vi "create temp folder.vi"(8 "error in":errorcluster, 9 "Temp?":bool, 11 "Path in":path) -> (0 "error out":errorcluster, 3 "Path out":path)   [LabVIEW 2023, in "User Interface.lvlib"]
uses:
  User Interface.lvlib
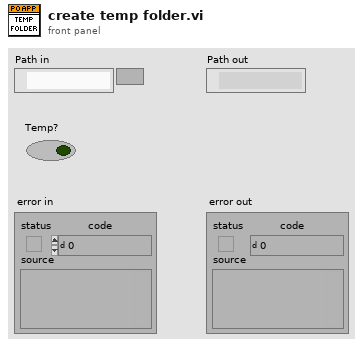
[diagram p1: front panel]
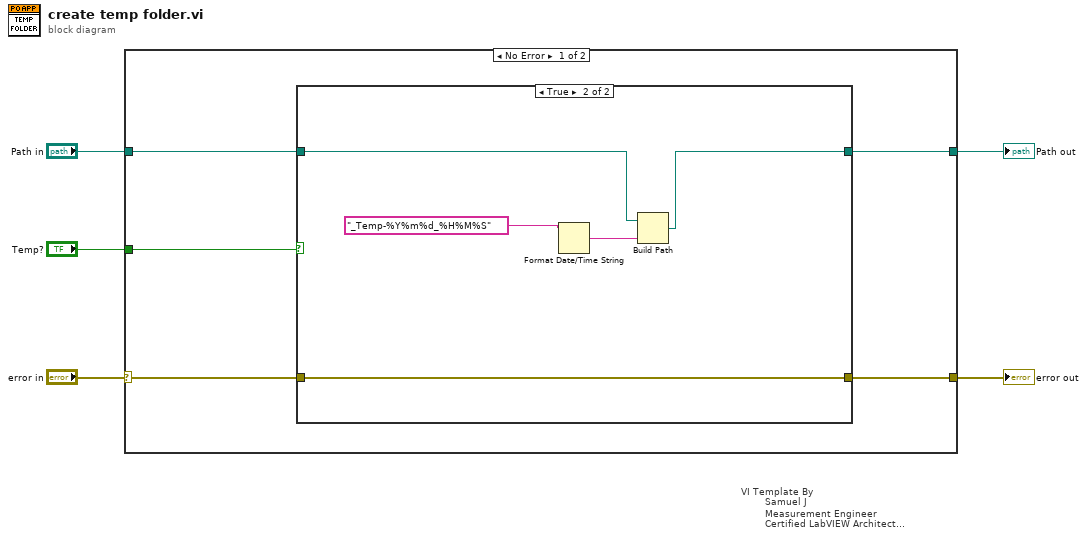
[diagram p0: block diagram]
diagram:
  n1 = case "VI Template By\n        Samuel J\n        Measurement Engineer\n        Certified LabVIEW Architect\n        Vestas Technology R&D Chennai" shown="No Error" "error in" {
    selector: "error in" -> [w6 w19]
    tunnel: [w7 w19] -> w4
    tunnel: "Path in" -> [w8 w18]
    tunnel: [w9 w18] -> w2
    tunnel: "Temp?" -> [w10 _]
    frame No Error {
      n2 = case shown="True" w10 {
        tunnel: [w12 w13] -> w9
        tunnel: w8 -> [w12 w17]
        tunnel: [w11 w16] -> w7
        tunnel: w6 -> [w11 w16]
        frame False {
        }
        frame True {
          n3 = Format Date/Time String(time format string (%c)="_Temp-%Y%m%d_%H%M%S") -> (date/time string=w14:string)  [unwired: 2 in]
          n4 = Build Path(base path=w17, name or relative path=w14) -> (appended path=w13:path)
        }
      }
    }
    frame Error {
    }
  }
  "error out" <- w4
  "Path out" <- w2
